vi "Check-storage-conditions.vi"(8 "error in (no error)":errorcluster, 11 "Data ref. in":refnum<data-value>) -> (0 "error out":errorcluster, 3 "Data ref.":refnum<data-value>, 5 "Passed?":bool)   [LabVIEW 2013, in "CameraVision.lvlib" / "CV-Main.lvclass"]
uses:
  CV-Main.lvclass
  UI/Popup-messages.ctl
  CV-Main.lvclass/CV-Main.ctl
  Storage/CV-Storage.lvclass/CV-Storage.ctl
  Read Acquis params.vi
  Read Analysis params.vi
  Read Config params.vi
  Read Correct params.vi
  Read Filter params.vi
  Read Mapping params.vi
  Read Temperature params.vi
  Read Storage params.vi
  Storage/Read Save what.vi
  Acquisition/CV-Acquisition.lvclass
  Analysis/CV-Analysis.lvclass
  Configuration/CV-Configuration.lvclass
  Correction/CV-Correction.lvclass
  Filter/CV-Filter.lvclass
  Mapping/CV-Mapping.lvclass
  Temperature/CV-Temperature.lvclass
  Storage/CV-Storage.lvclass
  UI/CV-UI.lvclass
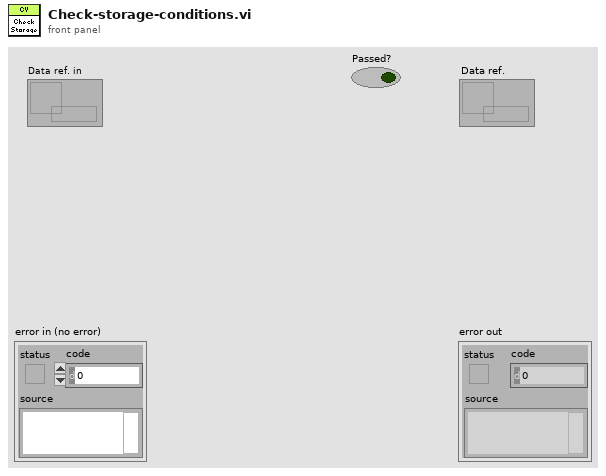
[diagram p1: front panel]
types:
  T1 = typedef "CameraVision.lvlib/CV-UI.lvclass/Popup-messages.ctl" = enum16{"Error-Black image", "Error-Camera config file", "Error-Camera connect", "Error-Grabber init", "Error-Camera setting", "Error-Image offset", "Error-Image import", "Error-Settings file not exist", "Error-Timing source", "Conflict-Filters", "Conflict-Map", "Conflict-Framerate", "Conflict-Charact", "Conflict-Temperature field", "Conflict-Temperature value", "Conflict-Storage-Binary image", "Conflict-Storage-Corrected image", "Conflict-Storage-Map", "Conflict-Storage-Charact", "Conflict-Storage-Temperature field", "Conflict-Storage-Temperature value", "Warning-File exist", "Warning-Parameter reset", "Warning-User cancel", "Info-Images imported"}
  T2 = cluster{"Original":bool, "Corrected":bool, "Binary":bool, "Temperature":bool, "Characteristics":bool, "Mapping":bool, "TemperatureValues":bool}
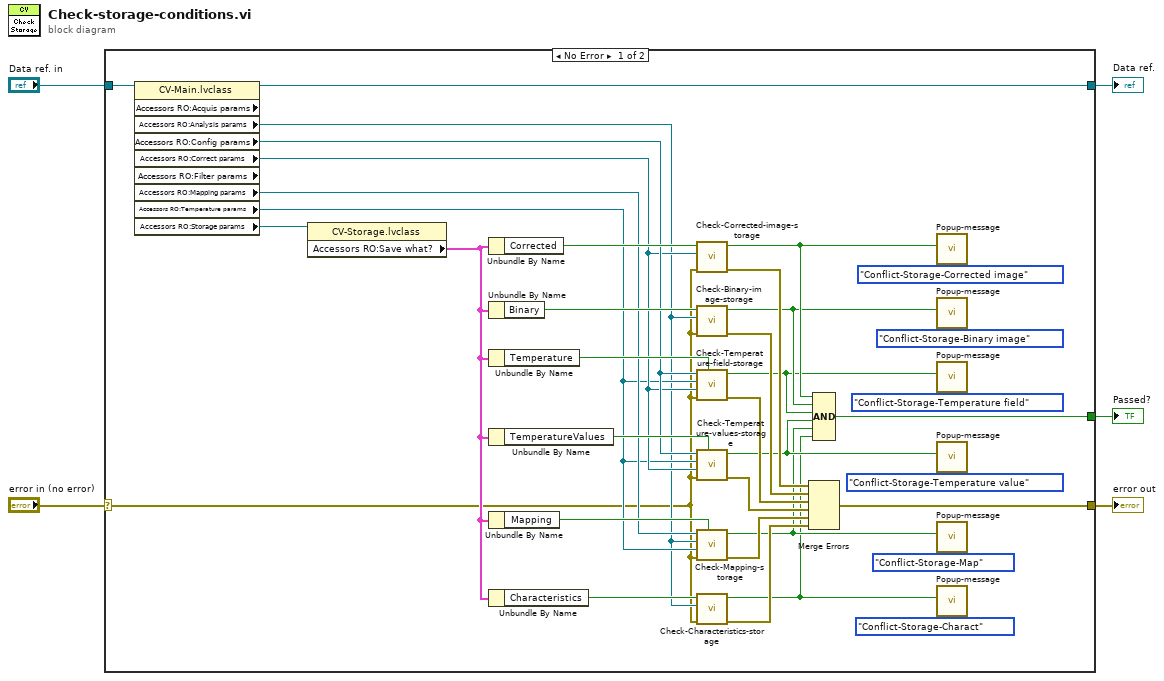
[diagram p0: block diagram]
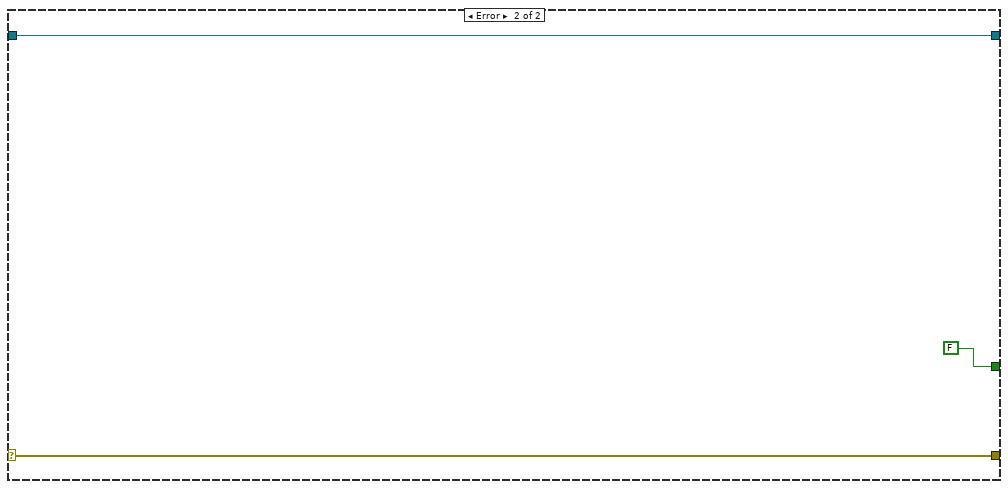
[diagram p2: hidden frame]
diagram:
  n1 = case shown="No Error" "error in (no error)" {
    selector: "error in (no error)" -> [w24 w44]
    tunnel: [w28 w44] -> w4
    tunnel: "Data ref. in" -> [w26 w43]
    tunnel: [w25 w43] -> w2
    tunnel: [w27 FALSE] -> w1
    frame No Error {
      n2 = property class="CV-Main.lvclass" props=["Accessors RO:Acquis params", "Accessors RO:Analysis params", "Accessors RO:Config params", "Accessors RO:Correct params", "Accessors RO:Filter params", "Accessors RO:Mapping params", "Accessors RO:Temperature params", "Accessors RO:Storage params"](reference=w26) -> (reference out=w25:refnum<data-value>, "Accessors RO:Analysis params"=w29:refnum<data-value>, "Accessors RO:Config params"=w33:refnum<data-value>, "Accessors RO:Correct params"=w32:refnum<data-value>, "Accessors RO:Mapping params"=w31:refnum<data-value>, "Accessors RO:Temperature params"=w30:refnum<data-value>, "Accessors RO:Storage params"=w34:refnum<data-value>)  [unwired: 1 in, 3 out]
      n3 = property class="CV-Storage.lvclass"(reference=w34) -> ("Accessors RO:Save what?"=w35:T2)  [unwired: 1 in, 2 out]
      n4 = Unbundle By Name(w35) -> ("Corrected"=w41:bool)
      n5 = Unbundle By Name(w35) -> ("Binary"=w40:bool)
      n6 = Unbundle By Name(w35) -> ("Temperature"=w39:bool)
      n7 = Unbundle By Name(w35) -> ("TemperatureValues"=w38:bool)
      n8 = Unbundle By Name(w35) -> ("Mapping"=w37:bool)
      n9 = Unbundle By Name(w35) -> ("Characteristics"=w36:bool)
      n10 = call "Check-Corrected-image-storage.vi"("error in"=w24, "Correct. params. ref."=w32, "Save?"=w41) -> ("error IO"=w23:errorcluster, "Passed?"=w16:bool)  [unwired: 7 in]
      n11 = call "Check-Binary-image-storage.vi"("error in"=w24, "Analysis params. ref."=w29, "Save?"=w40) -> ("error IO"=w22:errorcluster, "Passed?"=w14:bool)  [unwired: 7 in]
      n12 = call "Check-Temperature-field-storage.vi"("Save?"=w39, "error in"=w24, "Correct. params. ref."=w32, "Temp. params. ref."=w30, "Config. params. ref."=w33) -> ("error IO"=w21:errorcluster, "Passed?"=w13:bool)  [unwired: 5 in]
      n13 = call "Check-Temperature-values-storage.vi"("Save?"=w38, "error in"=w24, "Correct. params. ref."=w32, "Temp. params. ref."=w30, "Config. params. ref."=w33) -> ("error IO"=w20:errorcluster, "Passed?"=w10:bool)  [unwired: 5 in]
      n14 = call "Check-Mapping-storage.vi"("Save?"=w37, "error in"=w24, "Temp. params. ref."=w30, "Analysis params. ref."=w29, "Mapping params. ref."=w31) -> ("error IO"=w19:errorcluster, "Passed?"=w9:bool)  [unwired: 5 in]
      n15 = call "Check-Characteristics-storage.vi"("error in"=w24, "Analysis params. ref."=w29, "Save?"=w36) -> ("error IO"=w18:errorcluster, "Passed?"=w6:bool)  [unwired: 7 in]
      n16 = Merge Errors(w23, w22, w21, w20, w19, w18) -> (w28:errorcluster)
      n17 = Compound Arithmetic op=AND(w16, w14, w13, w10, w9, w6) -> (w27:bool)
      n18 = call "Popup-message.vi"("Message"=Popup-messages."Conflict-Storage-Corrected image", "Ignore?"=w16) -> ()  [unwired: 9 in, 1 out]
      n19 = call "Popup-message.vi"("Message"=Popup-messages."Conflict-Storage-Binary image", "Ignore?"=w14) -> ()  [unwired: 9 in, 1 out]
      n20 = call "Popup-message.vi"("Message"=Popup-messages."Conflict-Storage-Temperature field", "Ignore?"=w13) -> ()  [unwired: 9 in, 1 out]
      n21 = call "Popup-message.vi"("Message"=Popup-messages."Conflict-Storage-Temperature value", "Ignore?"=w10) -> ()  [unwired: 9 in, 1 out]
      n22 = call "Popup-message.vi"("Message"=Popup-messages."Conflict-Storage-Map", "Ignore?"=w9) -> ()  [unwired: 9 in, 1 out]
      n23 = call "Popup-message.vi"("Message"=Popup-messages."Conflict-Storage-Charact", "Ignore?"=w6) -> ()  [unwired: 9 in, 1 out]
    }
    frame Error {
    }
  }
  "error out" <- w4
  "Data ref." <- w2
  "Passed?" <- w1
